vi "Host_Test.vi"() -> ()   [LabVIEW 2012]
uses:
  <vilib>/rvi/interface/nirviOpenFPGA/nirviOpenFPGA.xnode
  <vilib>/rvi/interface/nirviReadWriteControl/nirviReadWriteControl.xnode
  <vilib>/rvi/interface/Simulation/niFpgaSimulationCallBeginRW.vi
  <vilib>/rvi/errors/niLvFpgaAdjustHostInterfaceError.vi
  <vilib>/rvi/interface/nirviMethod/nirviMethod.xnode
  <vilib>/rvi/interface/nirviCloseFPGA/nirviCloseFPGA.xnode
  <vilib>/FPGAPlugInAG/Dynamic/niLvFpga_Close_Dynamic.vi
  FPGA VIs/ResonanceScanner.vi
  <vilib>/FPGAPlugInAG/PXIe-7962R/niLvFpga_Open_PXIe-7962R.vi
  <vilib>/rvi/interface/common/dynamic/niFpgaDynamicAddResources.vi
  <vilib>/FPGAPlugInAG/Dynamic/niLvFpga_ReadFifo_Dynamic.vi
  <vilib>/rvi/errors/niLvFpgaMergeErrorWithErrorCode.vi
panel:
  out "Pixel Finished?":bool
  out "ToHostCh1FIFO Overflow":bool
  out "InterloopFIFO Timout":bool
  out "Resonance Scanner Trigger":bool
  out "Acquiring?":bool
  in  "stop":bool
  in  "Baseline16 Ch1":u16
  in  "Requested Pixels":u32
  out "Resonance Trigger":u32[](graph)
  in  "Samples per pixel":u32
  out "error out":errorcluster
  out "InterloopFIFO Overflow":bool
  out "ToHostCh1FIFO Overflow":bool
  out "Configured?":bool
  out "IO Module\\AI Over Range":bool
  out "Ch1":u32[](graph)
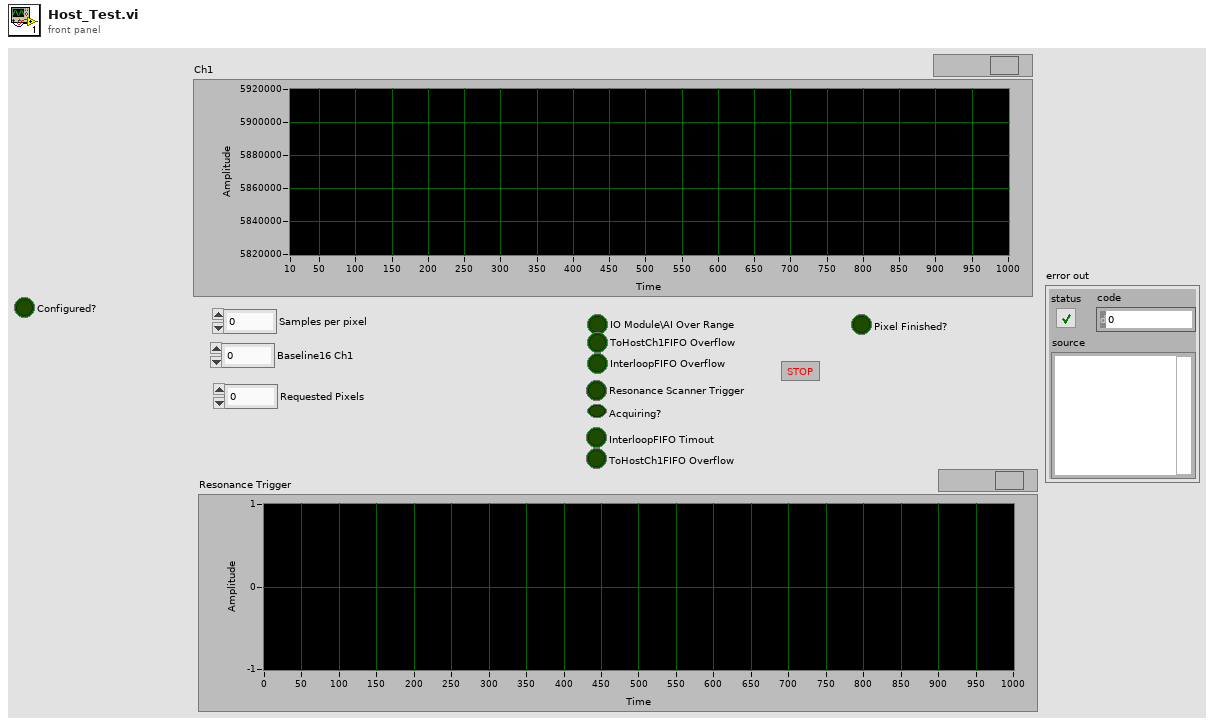
[diagram p1: front panel]
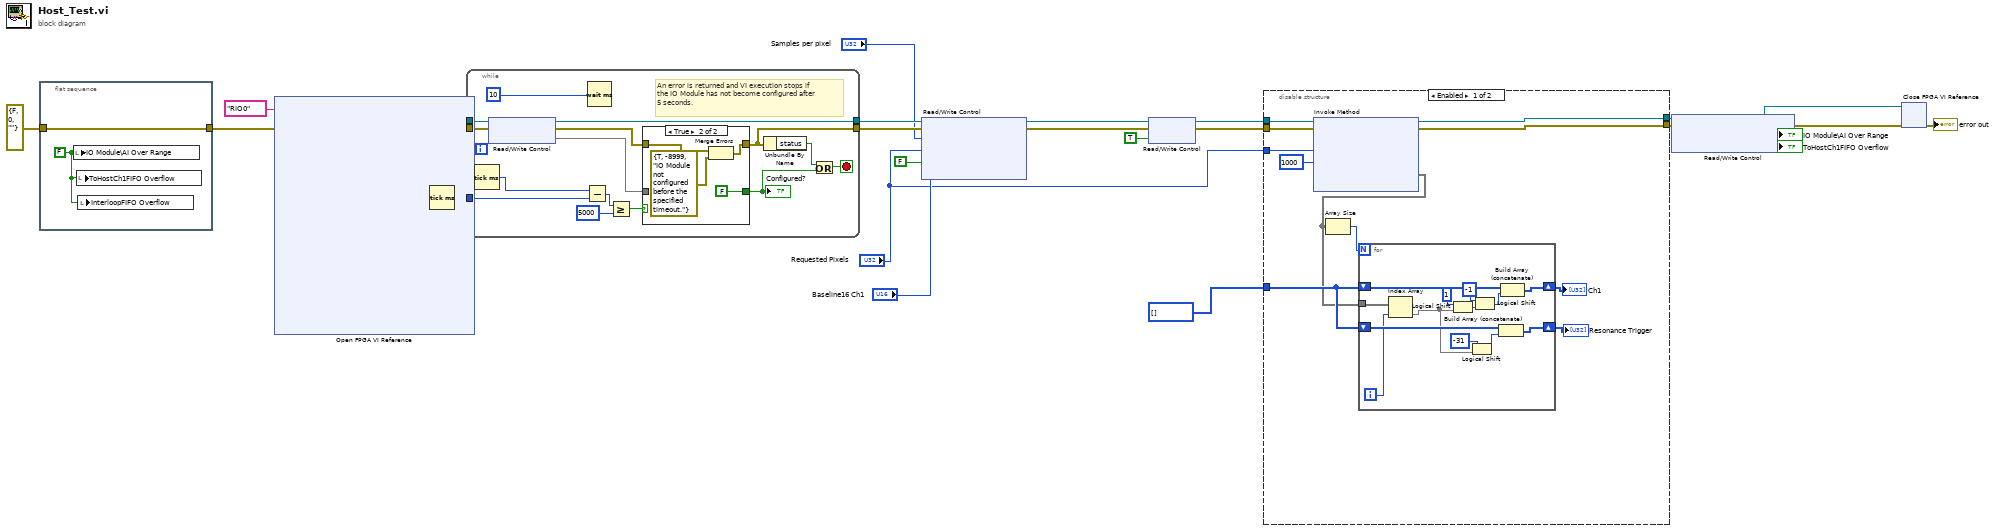
[diagram p0: block diagram]
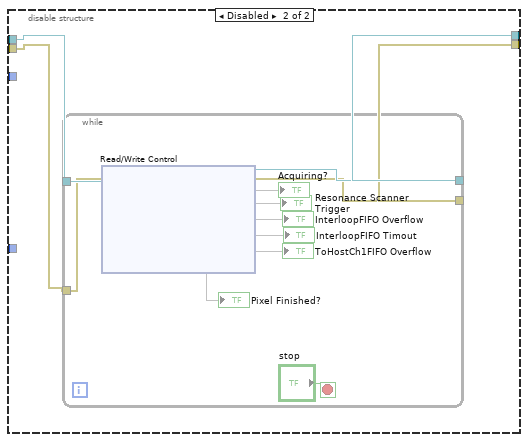
[diagram p2: hidden frame]
diagram:
  n1 = flat-sequence {
    tunnel: errorcluster {"status"=FALSE, "code"=0, "source"=""} ("error in") -> [w26]
    tunnel: [w26] -> w8
    frame #0 {
      w27 = FALSE ("IO Module\\AI Over Range")
      n2 = local write "IO Module\\AI Over Range"(w27) -> ()
      n3 = local write "ToHostCh1FIFO Overflow"(w27) -> ()
      n4 = local write "InterloopFIFO Overflow"(w27) -> ()
    }
  }
  n5 = xnode "Open FPGA VI Reference"("error in"=w8, "resource name"=tag "RIO0") -> ("FPGA VI Reference Out"=w14:refnum<k20>, "error out"=w15:errorcluster)
  n6 = Tick Count (ms)() -> (millisecond timer value=w13:u32)
  n7 = while {
    tunnel: w15 -> [w35]
    tunnel: [w39] -> w12
    tunnel: [w31] -> w11
    tunnel: w14 -> [w34]
    tunnel: w13 -> [w29]
    stop <- w37 stop-if-true
    # "An error is returned and VI execution stops if the IO Module has not become configured after 5 seconds."
    n8 = Tick Count (ms)() -> (millisecond timer value=w30:u32)
    n9 = xnode "Read/Write Control"("FPGA VI Reference In"=w34, "error in"=w35) -> ("FPGA VI Reference Out"=w31:refnum<k20>, "error out"=w32:errorcluster, "Configured?"=w33)
    n10 = Subtract(x=w30, y=w29) -> (x-y=w28:u32)
    n11 = Wait (ms)(milliseconds to wait=u32 10) -> ()  [unwired: 1 out]
    n12 = Greater Or Equal?(x=w28, y=u32 5000) -> (x >= y?=w40:bool)
    n13 = case shown="True" w40 {
      tunnel: [w44 FALSE ("Configured?")] -> w36
      tunnel: w33 -> [w44 _]
      tunnel: [w43 w47] -> w39
      tunnel: w32 -> [w43 w45]
      frame False {
      }
      frame True {
        n14 = Merge Errors(w45, errorcluster {"status"=TRUE, "code"=-8999, "source"="IO Module not configured before the specified timeout."} ("error in")) -> (w47:errorcluster)
      }
    }
    "Configured?" <- w36
    n15 = Unbundle By Name(w39) -> ("status"=w38:bool)
    n16 = Or(x=w38, y=w36) -> (x .or. y?=w37:bool)
  }
  n17 = xnode "Read/Write Control"("FPGA VI Reference In"=w11, "error in"=w12, "Samples per pixel"="Samples per pixel", "Requested pixels"="Requested Pixels", "Acquire continuously"=FALSE, "Baselinex8 Ch1"="Baseline16 Ch1") -> ("FPGA VI Reference Out"=w2:refnum<k20>, "error out"=w3:errorcluster)
  n18 = xnode "Read/Write Control"("FPGA VI Reference In"=w2, "error in"=w3, "Acquire"=TRUE) -> ("FPGA VI Reference Out"=w22:refnum<k20>, "error out"=w21:errorcluster)
  n19 = disable-structure shown="Enabled" {
    disable-tunnel: w22 -> [w59 w75]
    disable-tunnel: w21 -> [w58 w76]
    disable-tunnel: [w56 w74] -> w20
    disable-tunnel: [w55 w73] -> w18
    disable-tunnel: "Requested Pixels" -> [w54 _]
    disable-tunnel: u32[] [] -> [w52 _]
    frame Enabled {
      n20 = xnode "Invoke Method"("FPGA VI Reference In"=w59, "error in"=w58, "Number of Elements"=w54, "Timeout (ms)"=1000) -> ("FPGA VI Reference Out"=w56:refnum<k20>, "error out"=w55:errorcluster, "Data"=w51:void[])  [unwired: 1 out]
      n21 = Array Size(array=w51) -> (size(s)=w53:i32)
      n22 = for {
        N: w53 -> [_]
        tunnel: w51 -> [w64]
        shift-right: [w61] -> w50
        shift-left: w52 -> [w72]
        shift-right: [w60] -> w49
        shift-left: w52 -> [w71]
        i -> [w63]
        n23 = Index Array(array=w64, index=w63) -> (element=w62)
        n24 = Logical Shift(y=i16 1, x=w62) -> (x << y=w66:i16)
        n25 = Logical Shift(y=i16 -31, x=w62) -> (x << y=w69:i16)
        n26 = Logical Shift(y=i16 -1, x=w66) -> (x << y=w65:i16)
        n27 = Build Array (concatenate)(w71, w69) -> (w60:u32[])
        n28 = Build Array (concatenate)(w72, w65) -> (w61:u32[])
      }
      "Ch1" <- w50
      "Resonance Trigger" <- w49
    }
    frame Disabled {
      n29 = while {
        tunnel: w76 -> [w83]
        tunnel: w75 -> [w84]
        tunnel: [w86] -> w74
        tunnel: [w79] -> w73
        stop <- "stop" stop-if-true
        n30 = xnode "Read/Write Control"("FPGA VI Reference In"=w84, "error in"=w83) -> ("FPGA VI Reference Out"=w86:refnum<k20>, "error out"=w79:errorcluster, "Acquiring"=→"Acquiring?", "Resonance Trigger"=→"Resonance Scanner Trigger", "InterloopFIFO Overflow"=→"InterloopFIFO Overflow", "InterloopFIFO Timeout"=→"InterloopFIFO Timout", "ToHostCh1FIFO Overflow"=→"ToHostCh1FIFO Overflow", "Pixel finished?"=→"Pixel Finished?")
      }
    }
  }
  n31 = xnode "Read/Write Control"("FPGA VI Reference In"=w20, "error in"=w18) -> ("FPGA VI Reference Out"=w19:refnum<k20>, "error out"=w17:errorcluster, "IO Module\\AI Over Range"=→"IO Module\\AI Over Range", "ToHostCh1FIFO Overflow"=→"ToHostCh1FIFO Overflow")
  n32 = xnode "Close FPGA VI Reference"("FPGA VI Reference In"=w19, "error in"=w17) -> ("error out"=→"error out":errorcluster)
